vi "SP_BreakDown_Detail.vi"(8 "error in (no error)":errorcluster) -> (0 "error out":errorcluster)   [LabVIEW 2017]
uses:
  <vilib>/Utility/error.llb/DialogType.ctl
  <vilib>/addons/database/Connection.llb/DB Tools Open Connec (Path).vi
  <vilib>/addons/database/Connection.llb/Conn Execute.vi
  <vilib>/addons/database/Recordset.llb/Rec Fetch Recordset Data (R).vi
  <vilib>/addons/database/Recordset.llb/Rec Destroy - Connection.vi
  <vilib>/addons/database/NI_Database_API.lvlib
panel:
  out "Station size":i32
  in  "Cancel Button - Archive":bool
  in  "Download 2":bool
  in  "Get Rport 2":bool
  in  "Manage 2":bool
  out "Table 2":string[][](array[string])
  out "Table":string[][](table)
  in  "Shift":string(combo)
  in  "Station":string(combo)
  in  "To Date":timestamp format="%<%Y-%m-%d>T"
  in  "From Date":timestamp format="%<%Y-%m-%d>T"
  in  "Stakeholder":string(combo)
  # "Breakdown Manage"
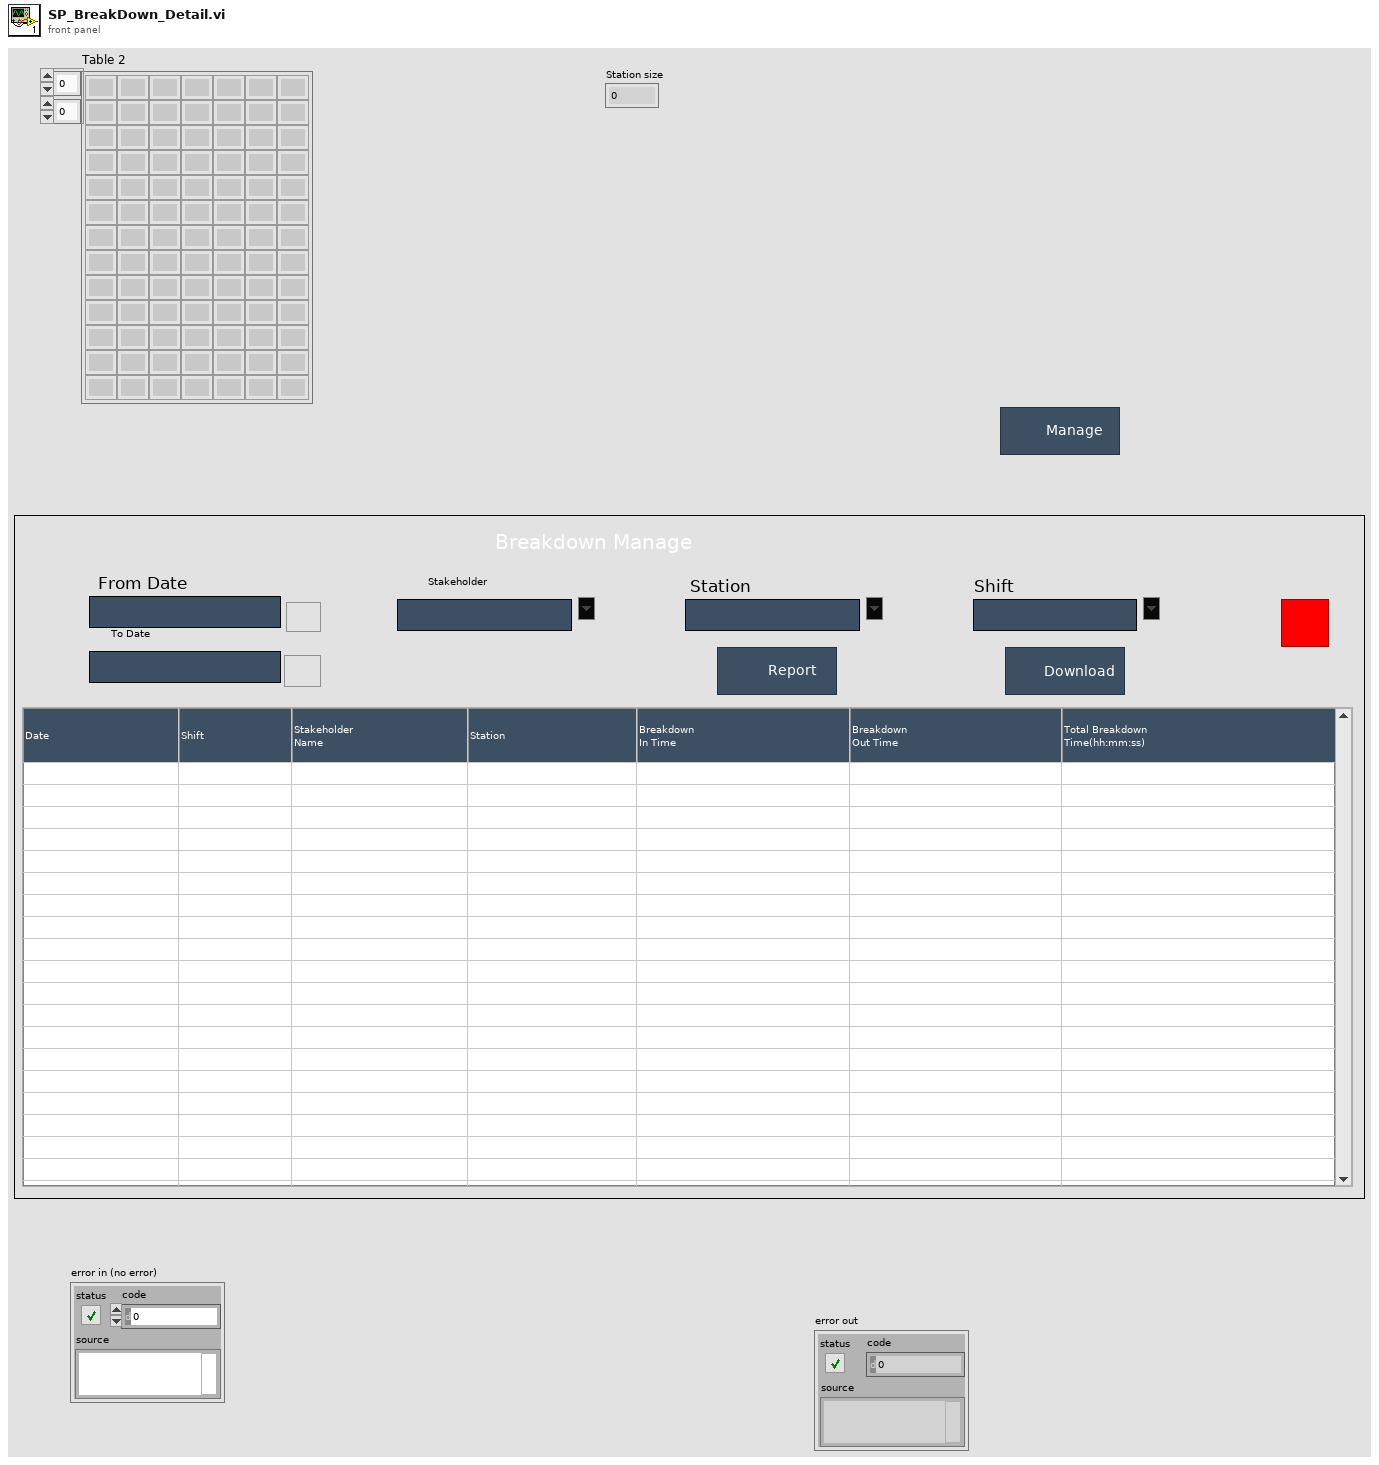
[diagram p1: front panel]
types:
  T1 = typedef "NI_Database_API.lvlib/Conn ObjectReference.ctl" = refnum<k1>
  T2 = typedef "NI_Database_API.lvlib/Rec ObjectReference.ctl" = refnum<k1>
  T3 = typedef "DialogType.ctl" = u16
  T4 = enum32{"invalid app kind", "Development System", "Run Time System", "Student Edition", "Embedded LabVIEW", "Evaluation", "Custom"}
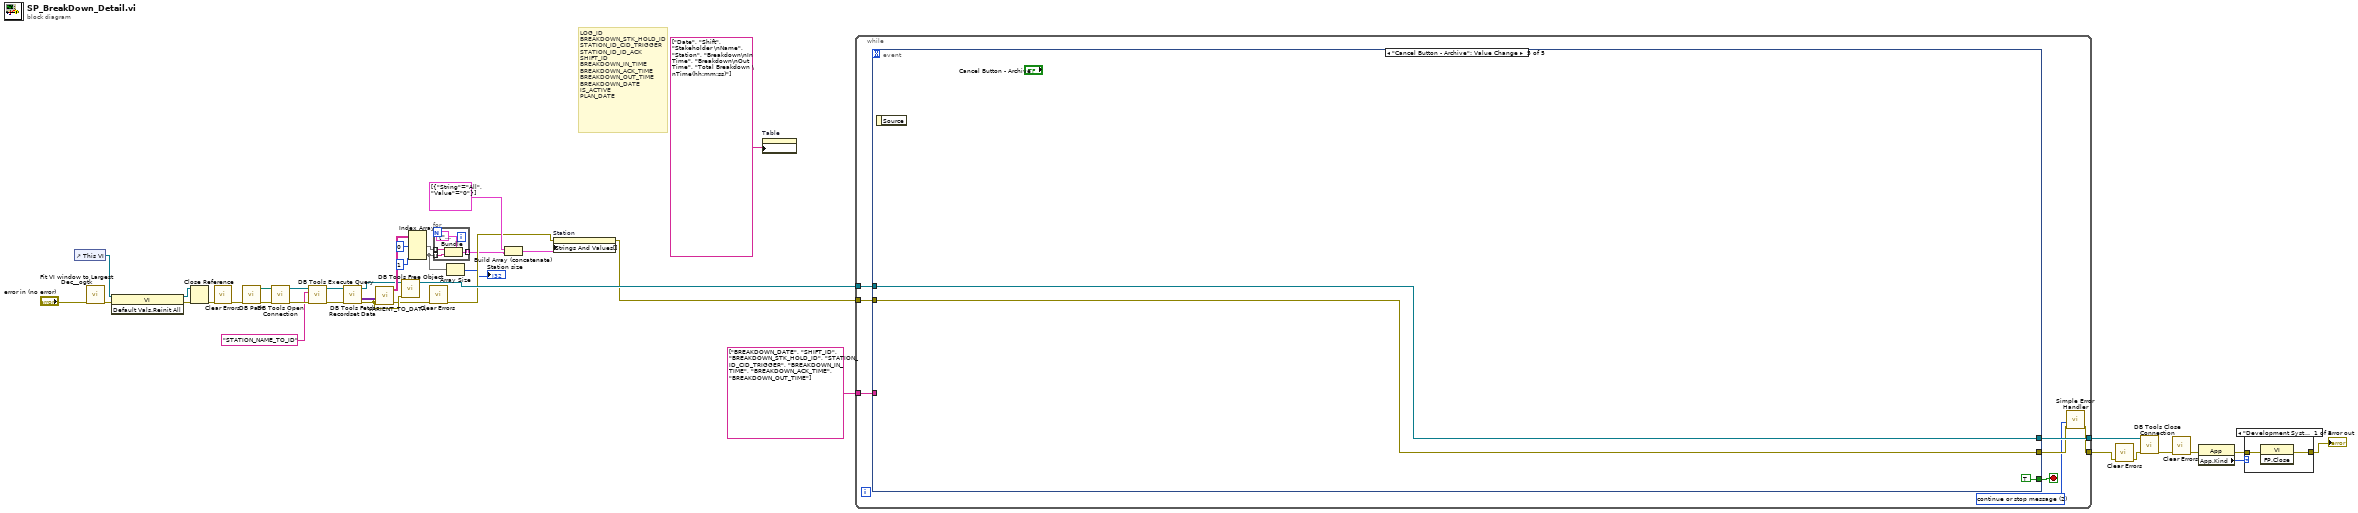
[diagram p0: block diagram]
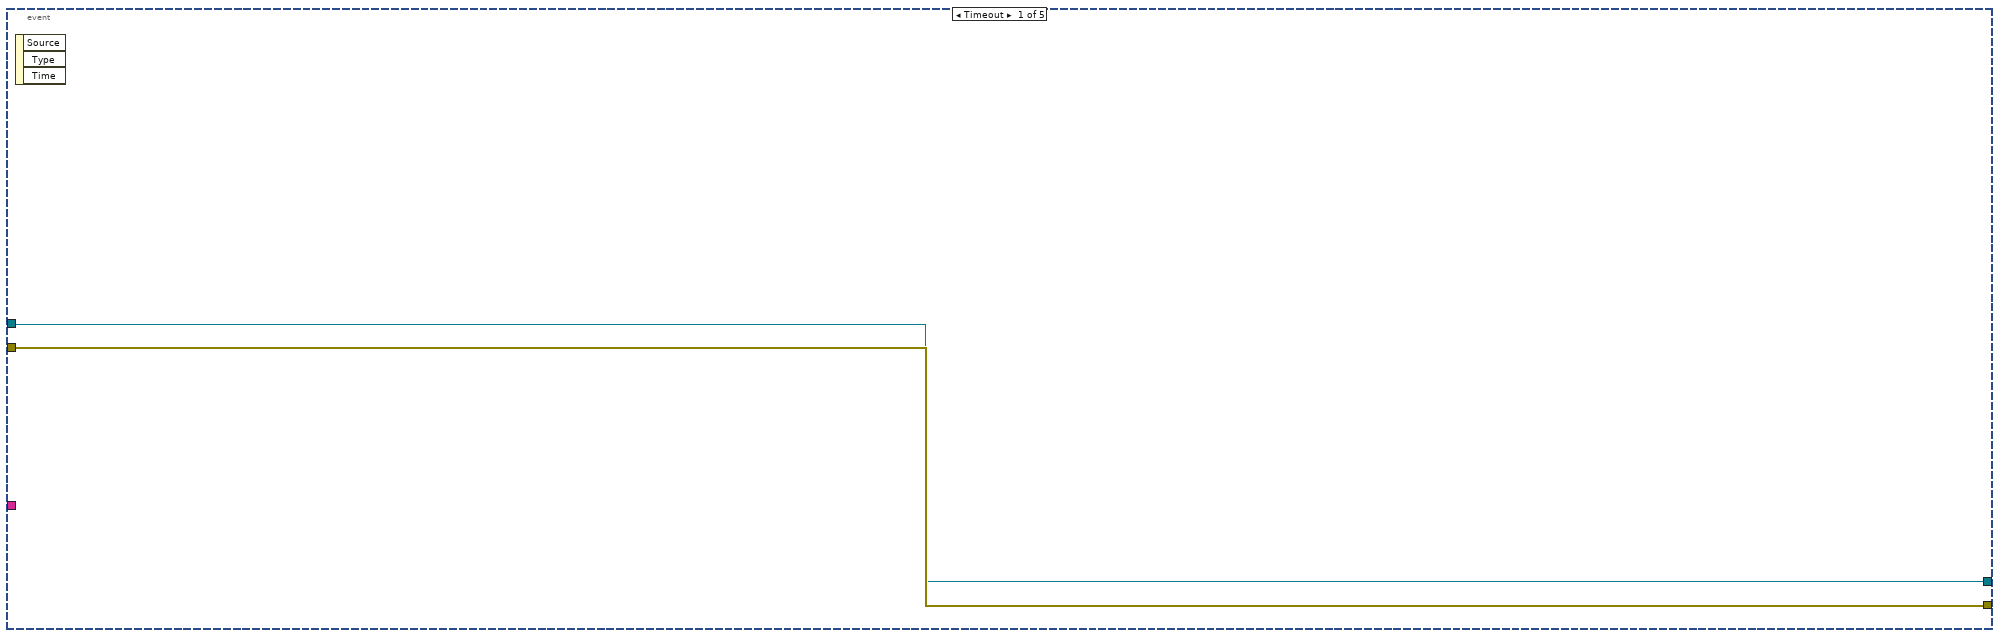
[diagram p2: hidden frame]
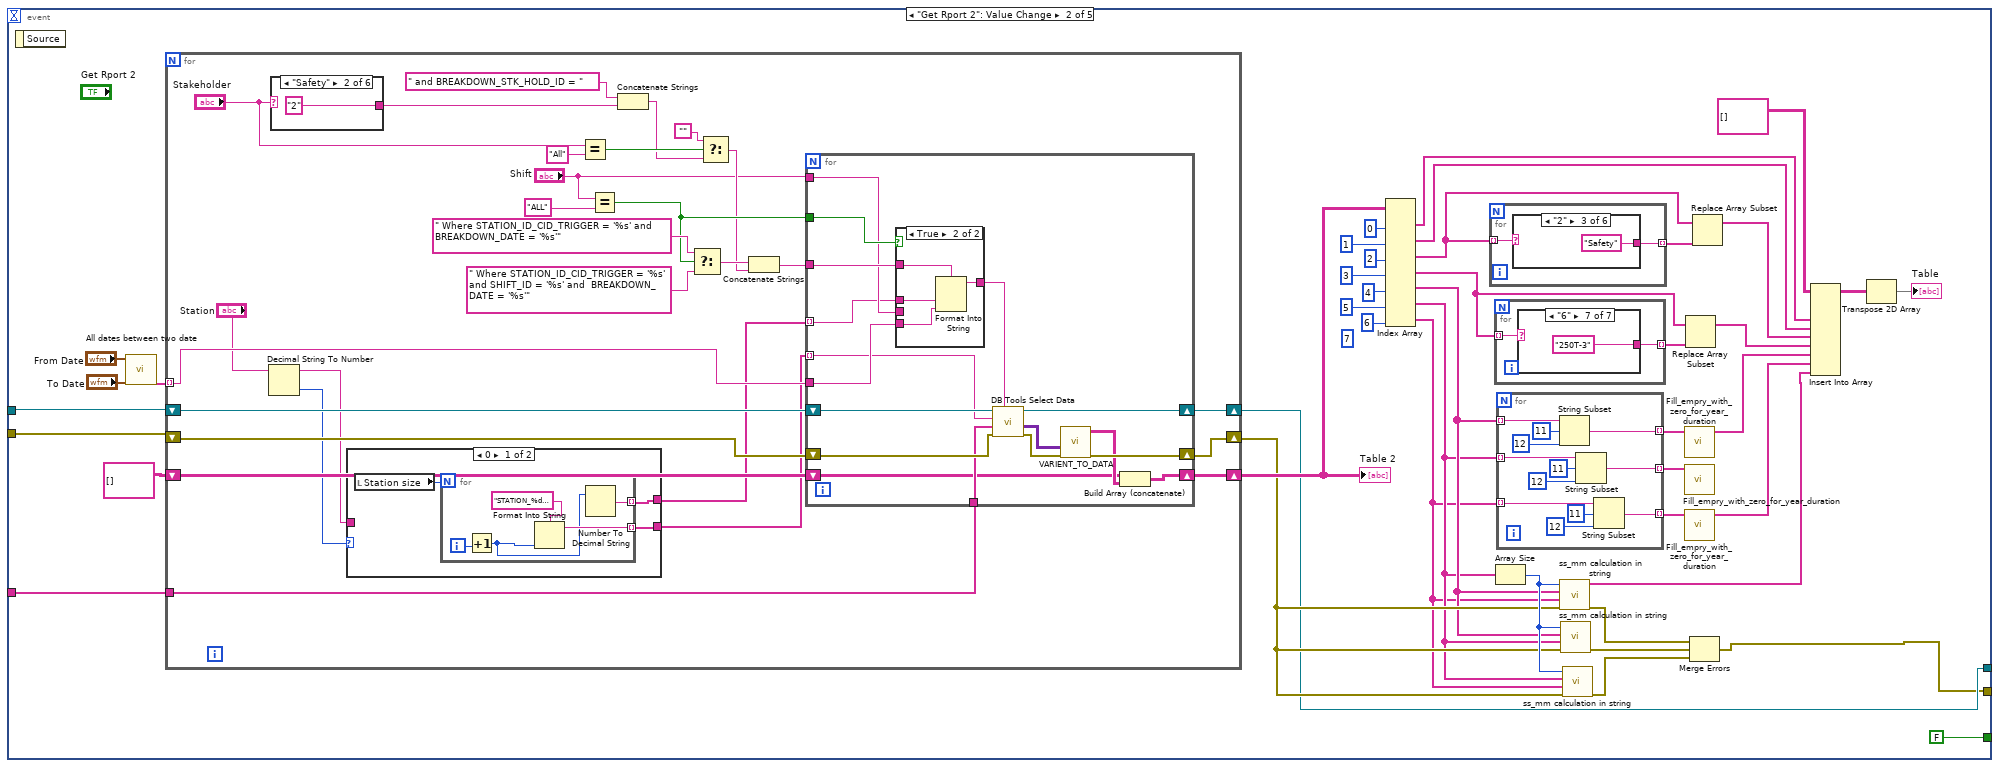
[diagram p3: hidden frame]
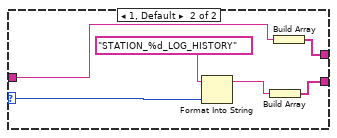
[diagram p4: hidden frame]
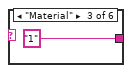
[diagram p6: hidden frame]
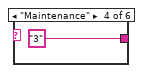
[diagram p7: hidden frame]
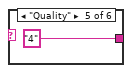
[diagram p8: hidden frame]
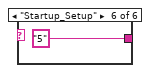
[diagram p9: hidden frame]
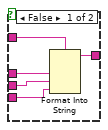
[diagram p10: hidden frame]
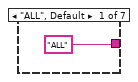
[diagram p11: hidden frame]
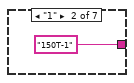
[diagram p12: hidden frame]
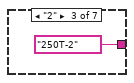
[diagram p13: hidden frame]
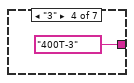
[diagram p14: hidden frame]
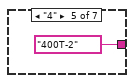
[diagram p15: hidden frame]
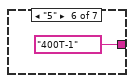
[diagram p16: hidden frame]
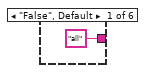
[diagram p17: hidden frame]
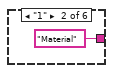
[diagram p18: hidden frame]
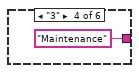
[diagram p19: hidden frame]
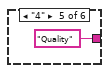
[diagram p20: hidden frame]
diagram:
  # "LOG_ID\nBREAKDOWN_STK_HOLD_ID\nSTATION_ID_CID_TRIGGER\nSTATION_ID_ID_ACK\nSHIFT_ID\nBREAKDOWN_IN_TIME\nBREAKDOWN_ACK_TIME\nBREAKDOWN_OUT_TIME\nBREAKDOWN_DATE\nIS_ACTIVE\nPLAN_DATE"
  n1 = control-ref of="This VI"() -> (w40:refnum<vi>)
  n2 = call <userlib>:"Fit VI window to Largest Dec__ogtk.vi"("error in (no error)"="error in (no error)") -> ("error out"=w32:errorcluster)  [unwired: 5 in, 1 out]
  n3 = invoke class="VI" method="Default Vals.Reinit All"(reference=w40, error in=w32) -> (reference out=w38:refnum<vi>, error out=w39:errorcluster)  [unwired: 1 in, 1 out]
  n4 = Close Reference(reference=w38, error in (no error)=w39) -> (error out=w2:errorcluster)
  n5 = call <vilib>:"Clear Errors.vi"("error in (no error)"=w2) -> ("error out"=w1:errorcluster)  [unwired: 5 in, 1 out]
  n6 = call "DB Path.vi"("error in"=w1) -> ("error out"=w37:errorcluster, "DB Path"=w36:path)  [unwired: 9 in]
  n7 = call-poly <vilib>:"DB Tools Open Connection.vi"("error in (no error)"=w37, "connection information"=w36) -> ("error out"=w13:errorcluster, "connection reference"=w15:T1)  [unwired: 6 in]
  n8 = call-poly <vilib>:"DB Tools Execute Query.vi"("error in (no error)"=w13, "SQL query"="STATION_NAME_TO_ID", "connection reference"=w15) -> ("error out"=w24:errorcluster, "recordset reference"=w25:T2)  [unwired: 5 in]
  n9 = call-poly <vilib>:"DB Tools Fetch Recordset Data.vi"("error in (no error)"=w24, "recordset reference"=w25) -> ("error out"=w19:errorcluster, "recordset data"=w23:variant[][], "recordset reference out"=w16:T2)  [unwired: 3 in]
  n10 = call "VARIENT_TO_DATA.vi"("data"=w23, "error in (no error)"=w19) -> ("Table"=w20:string[][], "error out"=w18:errorcluster)  [unwired: 7 in]
  n11 = call-poly <vilib>:"DB Tools Free Object.vi"("error in (no error)"=w19, "recordset reference"=w16) -> ("connection reference"=w14:T1)  [unwired: 8 in, 1 out]
  n12 = Index Array(array=w20, index (col) #1=0 ("index (row)"), index (col) #2=1 ("index (col)")) -> (element #1=w17:string[], element #2=w6:string[])  [unwired: 2 in]
  n13 = call <vilib>:"Clear Errors.vi"("error in (no error)"=w18) -> ("error out"=w9:errorcluster)  [unwired: 5 in, 1 out]
  n14 = for {
    tunnel: w17 -> [w44] mode=indexing
    tunnel: w6 -> [w43] mode=indexing
    tunnel: [w41] -> w7 mode=indexing
    n15 = Bundle(cluster=cluster{"String":string, "Value":string} {"String"="", "Value"=""}, "String"=w44, "Value"=w43) -> (w41:cluster{"String":string, "Value":string})
  }
  n16 = Array Size(array=w6) -> (size(s)=→"Station size":i32)
  n17 = Build Array (concatenate)(cluster{"String":string, "Value":string}[] [{"String"="All", "Value"="0"}] ("array"), w7) -> (w11:cluster{"String":string, "Value":string}[])
  n18 = property on="Station" class="CmbBox"(error in=w9, "Strings And Values[]"=w11) -> (error out=w8:errorcluster)  [unwired: 1 in, 1 out]
  n19 = property on="Table" class="Tbl (strict)"("Column Headers[]"=string[] ["Date", "Shift", "Stakeholder \nName", "Station", "Breakdown\nIn Time", "Breakdown\nOut Time", "Total Breakdown \nTime(hh:mm:ss)"] ("Column Header Strings[]")) -> ()  [unwired: 2 in, 2 out]
  n20 = while {
    tunnel: w14 -> [w52]
    tunnel: w8 -> [w51]
    tunnel: [w46] -> w4
    tunnel: [w50] -> w35
    tunnel: string[] ["BREAKDOWN_DATE", "SHIFT_ID", "BREAKDOWN_STK_HOLD_ID", "STATION_ID_CID_TRIGGER", "BREAKDOWN_IN_TIME", "BREAKDOWN_ACK_TIME", "BREAKDOWN_OUT_TIME"] -> [w49]
    stop <- w48 stop-if-true
    w45 = T3 2 items=["no dialog", "OK message", "continue or stop message", "OK message + warnings", "continue/stop + warnings"] ("type of dialog (OK msg:1)")
    n21 = event shown="[4] \"Cancel Button - Archive\": Value Change" {
      selector: _ -> [_ _ _ _ _]
      dyn-events: _ -> [_ _ _ _ _]
      timeout: _ -> [_ _ _ _ _]
      tunnel: w52 -> [w53 w74 w199 w202 w208]
      tunnel: w51 -> [w54 w73 w201 w206 w209]
      tunnel: [w54 w55 w200 w203 w209] -> w47
      tunnel: [w53 w75 w199 w202 w208] -> w50
      tunnel: w49 -> [_ w72 _ _ _]
      tunnel: [_ FALSE ("Cancel Button - Archive") _ _ TRUE] -> w48
      event Timeout {
        n22 = event-data() -> ()  [unwired: 1 in, 3 out]
      }
      event "Get Rport 2": Value Change {
        (unwired) 7 ("disabled index (col)")
        n23 = event-data() -> ()  [unwired: 1 in, 1 out]
        n24 = call "All dates between two date.vi"("To Date"="To Date", "From Date"="From Date") -> ("All Days (String)"=w71:string[])  [unwired: 8 in, 1 out]
        n25 = for {
          tunnel: w72 -> [w122]
          shift-right: [w117] -> w75
          shift-left: w74 -> [w124]
          shift-right: [w116] -> w76
          shift-left: w73 -> [w123]
          shift-right: [w114] -> w77
          shift-left: string[][] [] -> [w115]
          tunnel: w71 -> [w113] mode=indexing
          n26 = Decimal String To Number(string="Station") -> (number=w101:i32)  [unwired: 2 in, 1 out]
          n27 = case shown="\"Safety\"" "Stakeholder" {
            tunnel: [_ "2" "1" "3" "4" "5"] -> w109
            frame "All", Default {
            }
            frame "Safety" {
            }
            frame "Material" {
            }
            frame "Maintenance" {
            }
            frame "Quality" {
            }
            frame "Startup_Setup" {
            }
          }
          n28 = case shown="0" w101 {
            selector: w101 -> [_ w137]
            tunnel: [w127 w133] -> w98
            tunnel: "Station" -> [_ w136]
            tunnel: [w126 w135] -> w99
            frame 0 {
              n29 = local read "Station size"() -> (w125:i32)
              n30 = for {
                N: w125 -> [_]
                tunnel: [w130] -> w127 mode=indexing
                tunnel: [w128] -> w126 mode=indexing
                i -> [w131]
                n31 = Increment(x=w131) -> (x+1=w129:i32)
                n32 = Format Into String(format string="STATION_%d_LOG_HISTORY" ("table"), w129) -> (resulting string=w130:string)  [unwired: 2 in, 1 out]
                n33 = Number To Decimal String(number=w129) -> (decimal integer string=w128:string)  [unwired: 1 in]
              }
            }
            frame 1, Default {
              n34 = Format Into String(format string="STATION_%d_LOG_HISTORY" ("table"), w137) -> (resulting string=w134:string)  [unwired: 2 in, 1 out]
              n35 = Build Array(w134) -> (w133:string[])
              n36 = Build Array(w136) -> (w135:string[])
            }
          }
          n37 = Equal?(x="Stakeholder", y="All") -> (x = y?=w111:bool)
          n38 = Equal?(x="Shift", y="ALL" ("x")) -> (x = y?=w118:bool)
          n39 = Concatenate Strings(" and BREAKDOWN_STK_HOLD_ID = " ("format string"), w109) -> (w108:string)
          n40 = Select(t=" Where STATION_ID_CID_TRIGGER = '%s' and BREAKDOWN_DATE = '%s'" ("format string"), s=w118, f=" Where STATION_ID_CID_TRIGGER = '%s' and SHIFT_ID = '%s' and  BREAKDOWN_DATE = '%s'" ("format string")) -> (s? t:f=w106:string)
          n41 = Select(t="", s=w111, f=w108) -> (s? t:f=w105:string)
          n42 = Concatenate Strings(w106, w105) -> (w104:string)
          n43 = for {
            tunnel: w122 -> [w158]
            tunnel: w113 -> [w152]
            tunnel: w104 -> [w155]
            tunnel: w118 -> [w154]
            tunnel: w98 -> [w145] mode=indexing
            tunnel: "Shift" -> [w153]
            shift-right: [w150] -> w116
            shift-left: w123 -> [w159]
            shift-right: [w149] -> w117
            shift-left: w124 -> [w160]
            shift-right: [w146] -> w114
            shift-left: w115 -> [w147]
            tunnel: w99 -> [w144] mode=indexing
            n44 = case shown="True" w154 {
              tunnel: w155 -> [w165 w169]
              tunnel: w144 -> [w164 w168]
              tunnel: w153 -> [w162 _]
              tunnel: w152 -> [w161 w166]
              tunnel: [w163 w167] -> w151
              frame False {
                n45 = Format Into String(format string=w165, w164, w162, w161) -> (resulting string=w163:string)  [unwired: 2 in, 1 out]
              }
              frame True {
                n46 = Format Into String(format string=w169, w168, w166) -> (resulting string=w167:string)  [unwired: 2 in, 1 out]
              }
            }
            n47 = call <vilib>:"DB Tools Select Data.vi"("condition"=w151, "error in (no error)"=w159, "columns"=w158, "table"=w145, "connection reference"=w160) -> ("error out"=w156:errorcluster, "data"=w157:variant[][], "connection reference out"=w149:T1)  [unwired: 1 in]
            n48 = call "VARIENT_TO_DATA.vi"("data"=w157, "error in (no error)"=w156) -> ("Table"=w148:string[][], "error out"=w150:errorcluster)  [unwired: 7 in]
            n49 = Build Array (concatenate)(w147, w148) -> (w146:string[][])
          }
        }
        "Table 2" <- w77
        n50 = Index Array(array=w77, index (col) #1=0 ("disabled index (col)"), index (col) #2=1 ("disabled index (col)"), index (col) #3=2 ("disabled index (col)"), index (col) #4=3 ("disabled index (col)"), index (col) #5=4 ("disabled index (col)"), index (col) #6=5 ("disabled index (col)"), index (col) #7=6 ("disabled index (col)")) -> (element #1=w67:string[], element #2=w66:string[], element #3=w64:string[], element #4=w63:string[], element #5=w61:string[], element #6=w60:string[], element #7=w59:string[])  [unwired: 7 in]
        n51 = for {
          tunnel: w64 -> [w192] mode=indexing
          tunnel: [w191] -> w95 mode=indexing
          n52 = case shown="\"2\"" w192 {
            tunnel: ["all" "Material" "Safety" "Maintenance" "Quality" "Startup_Setup"] -> w191
            frame "False", Default {
            }
            frame "1" {
            }
            frame "2" {
            }
            frame "3" {
            }
            frame "4" {
            }
            frame "5" {
            }
          }
        }
        n53 = for {
          tunnel: w63 -> [w183] mode=indexing
          tunnel: [w182] -> w93 mode=indexing
          n54 = case shown="\"6\"" w183 {
            tunnel: ["ALL" "150T-1" "250T-2" "400T-3" "400T-2" "400T-1" "250T-3"] -> w182
            frame "ALL", Default {
            }
            frame "1" {
            }
            frame "2" {
            }
            frame "3" {
            }
            frame "4" {
            }
            frame "5" {
            }
            frame "6" {
            }
          }
        }
        n55 = Array Size(array=w60) -> (size(s)=w85:i32)
        n56 = for {
          tunnel: w61 -> [w175] mode=indexing
          tunnel: w60 -> [w174] mode=indexing
          tunnel: w59 -> [w173] mode=indexing
          tunnel: [w172] -> w81 mode=indexing
          tunnel: [w171] -> w80 mode=indexing
          tunnel: [w170] -> w79 mode=indexing
          n57 = String Subset(string=w175, offset (0)=11, length (rest)=12 ("length (rest)")) -> (substring=w172:string)
          n58 = String Subset(string=w174, offset (0)=11, length (rest)=12 ("length (rest)")) -> (substring=w171:string)
          n59 = String Subset(string=w173, offset (0)=11, length (rest)=12 ("length (rest)")) -> (substring=w170:string)
        }
        n60 = call "ss_mm calculation in string.vi"("error in (no error)"=w76, "Table 2"=w59, "Table"=w61, "Numeric"=w85) -> ("error out"=w84:errorcluster, "Array 2"=w56:string[])  [unwired: 6 in]
        n61 = call "ss_mm calculation in string.vi"("error in (no error)"=w76, "Table 2"=w60, "Table"=w61, "Numeric"=w85) -> ("error out"=w83:errorcluster)  [unwired: 6 in, 1 out]
        n62 = call "ss_mm calculation in string.vi"("error in (no error)"=w76, "Table 2"=w59, "Table"=w60, "Numeric"=w85) -> ("error out"=w82:errorcluster)  [unwired: 6 in, 1 out]
        n63 = call "Fill_empry_with_zero_for_year_duration.vi"("duration In"=w81) -> ("duration out"=w58:string[])  [unwired: 10 in]
        n64 = call "Fill_empry_with_zero_for_year_duration.vi"("duration In"=w80) -> ()  [unwired: 10 in, 1 out]
        n65 = call "Fill_empry_with_zero_for_year_duration.vi"("duration In"=w79) -> ("duration out"=w57:string[])  [unwired: 10 in]
        n66 = Replace Array Subset(array=w63, new element=w93) -> (w62:string[])  [unwired: 1 in]
        n67 = Merge Errors(w84, w83, w82) -> (w55:errorcluster)
        n68 = Replace Array Subset(array=w64, new element=w95) -> (w65:string[])  [unwired: 1 in]
        n69 = Insert Into Array(array=string[][] [], new element #1=w67, new element #2=w66, new element #3=w65, new element #4=w62, new element #5=w58, new element #6=w57, new element #7=w56) -> (w87:string[][])  [unwired: 2 in]
        n70 = Transpose 2D Array(2D array=w87) -> (transposed array=→"Table":string[][])
      }
      event "Manage 2": Value Change {
        n71 = event-data() -> ()  [unwired: 1 in, 6 out]
        n72 = call "manage breakdown sub.vi"("error in (no error)"=w201) -> ("error out"=w200:errorcluster)  [unwired: 10 in]
      }
      event "Download 2": Value Change {
        n73 = event-data() -> ()  [unwired: 1 in, 1 out]
        n74 = local read "Table"() -> (w205:string[][])
        n75 = call "Download_Report_subvi.vi"("error in (no error)"=w206, "Value"=w205, "Column Header Strings[]"=string[][] [["Date", "Shift", "Stakeholder Name", "Station", "Breakdown In Time", "Breakdown Ack Time", "Breakdown Out Time", "STK Response Time(hh:mm:ss)", "STK Resolution Time(hh:mm:ss)", "Total Breakdown Time(hh:mm:ss)"]]) -> ("error out"=w203:errorcluster)  [unwired: 8 in]
      }
      event "Cancel Button - Archive": Value Change {
        n76 = event-data() -> ()  [unwired: 1 in, 1 out]
      }
    }
    n77 = call <vilib>:"Simple Error Handler.vi"("type of dialog (OK msg:1)"=w45, "error in (no error)"=w47) -> ("error out"=w46:errorcluster)  [unwired: 3 in, 4 out]
  }
  n78 = call <vilib>:"Clear Errors.vi"("error in (no error)"=w4) -> ("error out"=w3:errorcluster)  [unwired: 5 in, 1 out]
  n79 = call <vilib>:"DB Tools Close Connection.vi"("error in (no error)"=w3, "connection reference"=w35) -> ("error out"=w28:errorcluster)  [unwired: 5 in]
  n80 = call <vilib>:"Clear Errors.vi"("error in (no error)"=w28) -> ("error out"=w31:errorcluster)  [unwired: 5 in, 1 out]
  n81 = property class="App"(error in=w31) -> (error out=w30:errorcluster, "App.Kind"=w29:T4)  [unwired: 1 in, 1 out]
  n82 = case shown="\"Development System\", Default" w29 {
    tunnel: w30 -> [w210 w213]
    tunnel: [w211 w212] -> w27
    frame "Development System", Default {
      n83 = invoke class="VI" method="FP.Close"(error in=w210) -> (error out=w211:errorcluster)  [unwired: 2 in, 2 out]
    }
    frame "Run Time System" {
      n84 = invoke class="VI" method="FP.Close"(error in=w213) -> (error out=w212:errorcluster)  [unwired: 2 in, 2 out]
    }
  }
  "error out" <- w27
